vi "Interpolation_radial.vi"() -> ()   [LabVIEW 2013]
doc: "Illustrates how to use the Interpolate 2D Scattered VI to perform interpolation on scattered and grid data."
uses:
  <vilib>/Math Plots/3D Math Plots/3D Scatter/3D Scatter XCtrl/3D Scatter.xctl
  <vilib>/Math Plots/3D Math Plots/3D Surface/3D Surface XCtrl/3D Surface.xctl
  <vilib>/Analysis/1siggen.llb/Ramp Pattern by Samples.vi
  <vilib>/Math Plots/3D Math Plots/3D Scatter/3D Scatter Datatype/Public/Plot Helper (Vector).vi
  <vilib>/gmath/interp.llb/Create Mesh Grid (2D) (x,y arrays).vi
  <vilib>/gmath/interp.llb/Interpolate 2D Scattered (2D).vi
  <vilib>/Math Plots/3D Math Plots/3D Surface/3D Surface Datatype/Public/Plot Helper (Matrix).vi
  <vilib>/Utility/file.llb/Read From Spreadsheet File (DBL).vi
  <vilib>/Analysis/NI_AALBase.lvlib
  <vilib>/gmath/NI_AAL_Interpolation.lvlib
  <vilib>/gmath/NI_Gmath.lvlib
  <vilib>/Math Plots/3D Math Plots/3D Scatter/3D Scatter Datatype/3D Scatter Datatype.lvclass
  <vilib>/Math Plots/3D Math Plots/3D Surface/3D Surface Datatype/3D Surface Datatype.lvclass
panel:
  out "Zi":dbl[][](array[numeric])
  out "Raw Data 2":refnum<class "3D Plot Datatype.lvclass">[](xcontrol)
  out "all rows":dbl[][](array[numeric]) format="%0.3f"
  out "Waveform Graph":dbl[](graph)
  out "Interpolation":refnum<class "3D Plot Datatype.lvclass">[](xcontrol)
  out "Raw Data":refnum<class "3D Plot Datatype.lvclass">[](xcontrol)
  in  "Data":u16(ring) items=["Scattered Data", "Grid Data"]
  in  "Method":i32(ring)=1 items=["nearest", "linear", "cubic", "biharmonic spline "]
  # "Overview: Illustrates how to use the Interpolate 2D Scattered VI to perform interpolation on scattered and grid data.\nRequirements: LabVIEW Full Development System\nInstructions: \n1. Use the Data option to choose between scattered or grid data.\n2. Use the Method option to choose the interpolation method.\n3. Run the VI.\n4. Observe the difference in input data types and interpolation methods on the Raw Data and Interpolation graphs."
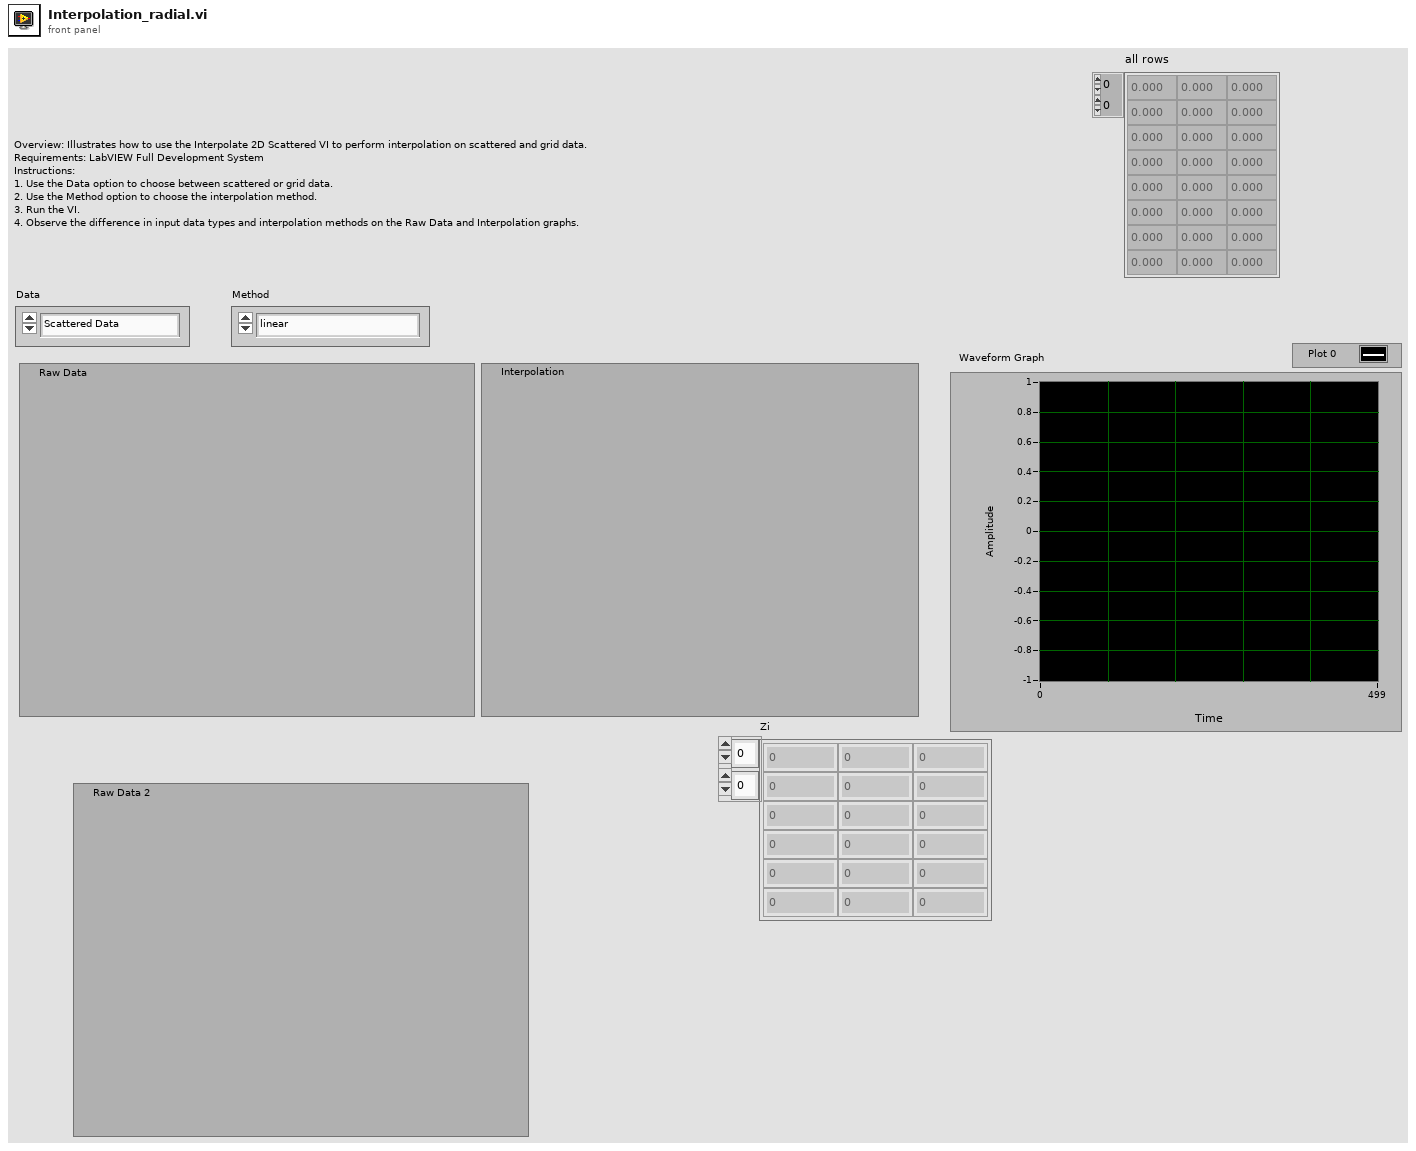
[diagram p1: front panel]
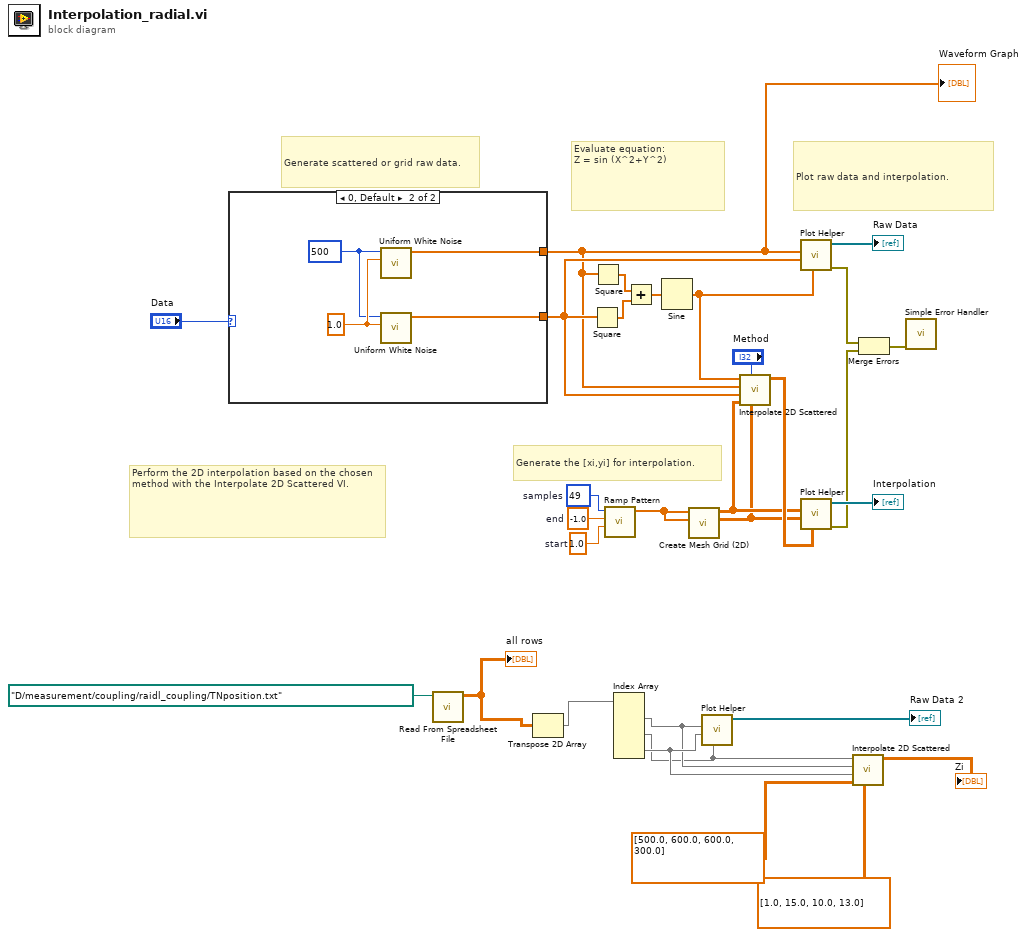
[diagram p0: block diagram]
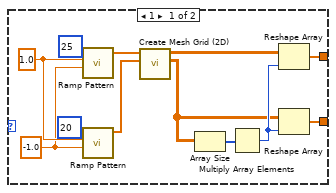
[diagram p2: hidden frame]
diagram:
  w23 = 1.0  # start
  w25 = 49  # samples
  w26 = -1.0  # end
  # "Generate the [xi,yi] for interpolation."
  # "Generate scattered or grid raw data."
  # "Perform the 2D interpolation based on the chosen method with the Interpolate 2D Scattered VI."
  # "Plot raw data and interpolation."
  # "Evaluate equation:\nZ = sin (X^2+Y^2)"
  n1 = case shown="0, Default" "Data" {
    tunnel: [w33 w43] -> w11
    tunnel: [w32 w44] -> w21
    frame 1 {
      w31 = -1.0 ("start")
      w41 = 1.0
      n2 = call-poly <vilib>:"Ramp Pattern.vi"("start"=w31, "end"=w41, "samples"=25) -> ("Ramp Pattern"=w40:dbl[])  [unwired: 7 in, 1 out]
      n3 = call-poly <vilib>:"Ramp Pattern.vi"("start"=w31, "end"=w41, "samples"=20) -> ("Ramp Pattern"=w39:dbl[])  [unwired: 7 in, 1 out]
      n4 = call-poly <vilib>:"Create Mesh Grid (2D).vi"("y domain"=w39, "x domain"=w40) -> ("Y"=w34:dbl[][], "X"=w37:dbl[][])  [unwired: 7 in, 1 out]
      n5 = Array Size(array=w34) -> (size(s)=w38:i32[])
      n6 = Multiply Array Elements(1:w38) -> (0:w36:i32)
      n7 = Reshape Array(w37, w36) -> (w33:dbl[])
      n8 = Reshape Array(w34, w36) -> (w32:dbl[])
    }
    frame 0, Default {
      w46 = 1.0
      w45 = 500 ("samples")
      n9 = call <vilib>:"Uniform White Noise.vi"("amplitude"=w46, "samples"=w45) -> ("uniform white noise"=w43:dbl[])  [unwired: 8 in, 1 out]
      n10 = call <vilib>:"Uniform White Noise.vi"("amplitude"=w46, "samples"=w45) -> ("uniform white noise"=w44:dbl[])  [unwired: 8 in, 1 out]
    }
  }
  "Waveform Graph" <- w11
  n11 = call-poly <vilib>:"Read From Spreadsheet File.vi"("file path (dialog if empty)"=path "D:/measurement/coupling/raidl_coupling/TNposition.txt") -> ("all rows"=w9:dbl[][])  [unwired: 6 in, 4 out]
  "all rows" <- w9
  n12 = Transpose 2D Array(2D array=w9) -> (transposed array=w8:dbl[][])
  n13 = Square(x=w21) -> (x^2=w30:dbl[])
  n14 = Square(x=w11) -> (x^2=w28:dbl[])
  n15 = call-poly <vilib>:"Ramp Pattern.vi"("start"=w23, "end"=w26, "samples"=w25) -> ("Ramp Pattern"=w24:dbl[])  [unwired: 7 in, 1 out]
  n16 = Index Array(array=w8) -> (element #1=w3:dbl[], element #2=w2:dbl[], element #3=w7:dbl[])  [unwired: 6 in]
  n17 = Add(x=w28, y=w30) -> (x+y=w29:dbl[])
  n18 = Sine(x=w29) -> (sin(x)=w20:dbl[])
  n19 = call-poly <vilib>:"Create Mesh Grid (2D).vi"("y domain"=w24, "x domain"=w24) -> ("Y"=w16:dbl[][], "X"=w17:dbl[][])  [unwired: 7 in, 1 out]
  n20 = call-poly <vilib>:"Plot Helper.vi"("z vector"=w2, "y vector"=w7, "x vector"=w3) -> ("3D Plot lvclass Array out"=→"Raw Data 2":refnum<class "3D Plot Datatype.lvclass">[])  [unwired: 3 in, 5 out]
  n21 = call-poly <vilib>:"Interpolate 2D Scattered.vi"("Yi"=w16, "method"="Method", "Xi"=w17, "Y"=w21, "X"=w11, "Z"=w20) -> ("Zi"=w18:dbl[][])  [unwired: 4 in, 1 out]
  n22 = call-poly <vilib>:"Plot Helper.vi"("z vector"=w20, "y vector"=w21, "x vector"=w11) -> ("error out"=w15:errorcluster, "3D Plot lvclass Array out"=→"Raw Data":refnum<class "3D Plot Datatype.lvclass">[])  [unwired: 3 in, 4 out]
  n23 = call-poly <vilib>:"Plot Helper.vi"("z matrix"=w18, "y matrix"=w16, "x matrix"=w17) -> ("error out"=w14:errorcluster, "3D Plot lvclass Array out"=→"Interpolation":refnum<class "3D Plot Datatype.lvclass">[])  [unwired: 3 in, 4 out]
  n24 = call-poly <vilib>:"Interpolate 2D Scattered.vi"("Yi"=dbl[][] [[1.0, 15.0], [10.0, 13.0]] ("Xi"), "Xi"=dbl[][] [[500.0, 600.0], [600.0, 300.0]], "Y"=w7, "X"=w3, "Z"=w2) -> ("Zi"=→"Zi":dbl[][])  [unwired: 5 in, 1 out]
  n25 = Merge Errors(w15, w14) -> (w13:errorcluster)
  n26 = call <vilib>:"Simple Error Handler.vi"("error in (no error)"=w13) -> ()  [unwired: 4 in, 5 out]
